vi "Merge Overlay With Image.vi"(6 "Image RGB":T1=refnum, 7 "ROI Cluster":T2={"left annulus"={"Center X"=929, "Center Y"=663, "Inner Radius"=200, "Outer Radius"=405, "Start Angle"=90.0, "End Angle"=180.0}, "right annulus"={"Center X"=929, "Center Y"=663, "Inner Radius"=200, "Outer Radius"=405, "Start Angle"=90.0, "End Angle"=180.0}, "Threshold Range"={"Lower value"=106.82432432432432, "Upper value"=255.0}, "[Avg BG]"=[0, 0, 0, 0, 0, 0, 0, 0, 0, 0, 0, 0, 0, 0, 0, 0, 0, 0, 0, 0, 0, 0, 0, 0, 0, 0, 0, 0, 0, 0, 0, 0], "Number of Sectors"=0, "Left ROI"={"Global Rectangle"=[], "Contours"=[]}, "Right ROI"={"Global Rectangle"=[], "Contours"=[]}, "Left Start Angle Duty Cycle"=0.0, "Left End Angle Duty Cycle"=0.0, "Right End Angle Duty Cycle"=0.0, "Right Start Angle Duty Cycle"=0.0, "[Sector ROIs]"=[], "Consecutive Sector Threshold"=0} {"[Sector ROIs]"."Contours"."Type" items=["No Selection", "Point", "Line", "Rectangle", "Oval", "Polygon", "Freehand Region", "Annulus", "Unused2", "Unused3", "Broken Line", "Freehand Line", "Rotated Rectangle"]; "Right ROI"."Contours"."Type" items=["No Selection", "Point", "Line", "Rectangle", "Oval", "Polygon", "Freehand Region", "Annulus", "Unused2", "Unused3", "Broken Line", "Freehand Line", "Rotated Rectangle"]; "Left ROI"."Contours"."Type" items=["No Selection", "Point", "Line", "Rectangle", "Oval", "Polygon", "Freehand Region", "Annulus", "Unused2", "Unused3", "Broken Line", "Freehand Line", "Rotated Rectangle"]; "Threshold Range"."Upper value" min=0.0 max=255.0 scale=0.0..255.0; "Threshold Range"."Lower value" min=0.0 max=255.0 scale=0.0..255.0; "right annulus"."End Angle" format="%.2f"; "right annulus"."Start Angle" format="%.2f"; "right annulus"."Center X" scale=0.0..1024.0; "left annulus"."End Angle" format="%.2f"; "left annulus"."Start Angle" format="%.2f"; "left annulus"."Center X" scale=0.0..1024.0}, 8 "Error in":errorcluster, 9 "Left Edge":u16, 10 "Right Edge":u16, 11 "Image In":T1=refnum) -> (0 "error out":errorcluster, 3 "Image Out":T1)   [LabVIEW 2013]
uses:
  <vilib>/vision/Image Controls.llb/IMAQ Image.ctl
  Image Processing/Mask ROI Cluster.ctl
  <vilib>/vision/NI_Vision_Development_Module.lvlib
  Common/Timing/Timing Lib.lvlib
panel:
  out "x-y":dbl
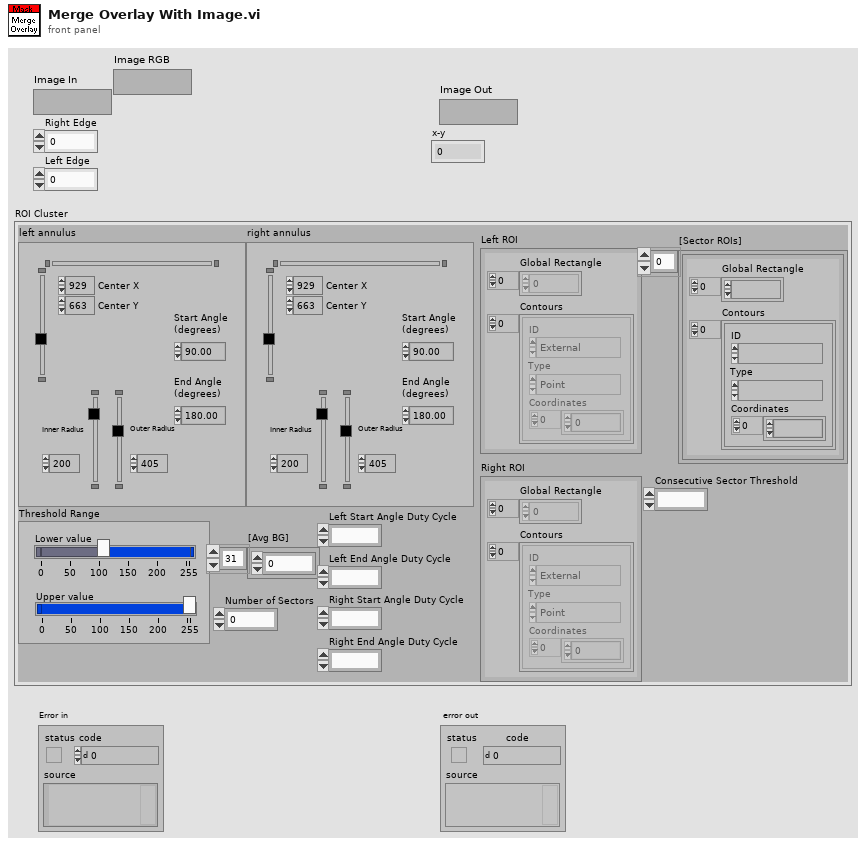
[diagram p1: front panel]
types:
  T1 = typedef "IMAQ Image.ctl" = refnum<image>
  T2 = typedef "Mask ROI Cluster.ctl" = cluster{"left annulus":T3, "right annulus":T3, "Threshold Range":cluster{"Lower value":dbl, "Upper value":dbl}, "[Avg BG]":u8[], "Number of Sectors":u8, "Left ROI":T4, "Right ROI":T4, "Left Start Angle Duty Cycle":fxp<+,8,0>, "Left End Angle Duty Cycle":fxp<+,8,0>, "Right End Angle Duty Cycle":fxp<+,8,0>, "Right Start Angle Duty Cycle":fxp<+,8,0>, "[Sector ROIs]":T4[], "Consecutive Sector Threshold":u8}
  T3 = typedef "IMAQ Circle" = cluster{"Center X":i32, "Center Y":i32, "Inner Radius":i32, "Outer Radius":i32, "Start Angle":dbl, "End Angle":dbl}
  T4 = typedef "ROI Descriptor" = cluster{"Global Rectangle":i32[], "Contours":cluster{"ID":enum32{"External", "Internal"}, "Type":u32, "Coordinates":i32[]}[]}
  T5 = typedef "Image Type" = u32
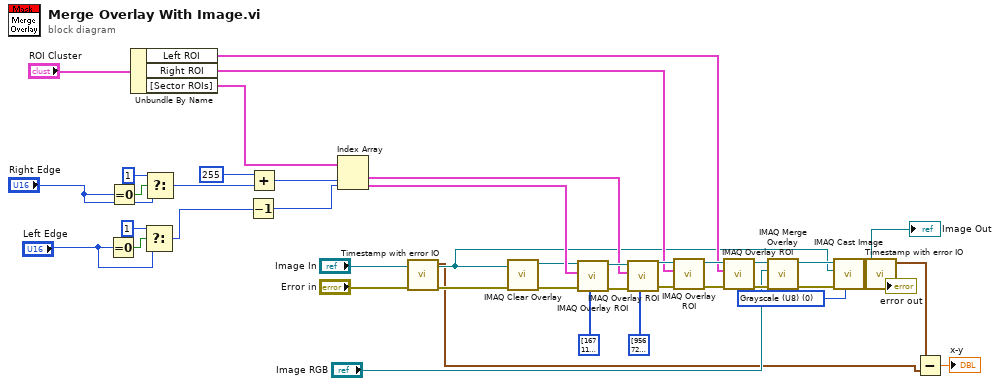
[diagram p0: block diagram]
diagram:
  w10 = T5 0 items=["Grayscale (U8)", "Grayscale (I16)", "Grayscale (SGL)", "Complex (CSG)", "RGB (U32)", "HSL (U32)", "RGB (U64)", "Grayscale (U16)"] ("Image Type")
  n1 = Equal To 0?(x="Left Edge") -> (x = 0?=w20:bool)
  n2 = Equal To 0?(x="Right Edge") -> (x = 0?=w22:bool)
  n3 = Unbundle By Name("ROI Cluster") -> ("Left ROI"=w31:T4, "Right ROI"=w30:T4, "[Sector ROIs]"=w29:T4[])
  n4 = Select(t=u16 1, s=w20, f="Left Edge") -> (s? t:f=w18:u16)
  n5 = Select(t=u16 1, s=w22, f="Right Edge") -> (s? t:f=w19:u16)
  n6 = Decrement(x=w18) -> (x-1=w38:u16)
  n7 = Add(x=u16 255, y=w19) -> (x+y=w39:u16)
  n8 = Index Array(array=w29, index #1=w39, index #2=w38) -> (element #1=w32:T4, element #2=w33:T4)
  n9 = call "Timestamp with error IO.vi"("error in (no error)"="Error in") -> ("error out"=w5:errorcluster, "current time"=w2:timestamp)  [unwired: 9 in]
  n10 = call "IMAQ Clear Overlay"("error in (no error)"=w5, "Image"="Image In") -> ("error out"=w26:errorcluster, "Image Out"=w27:T1)  [unwired: 8 in]
  n11 = call "IMAQ Overlay ROI"("Colors (Green)"=u32[] [16711935], "error in (no error)"=w26, "ROI Descriptor"=w33, "Image"=w27) -> ("error out"=w42:errorcluster, "Image Out"=w41:T1)  [unwired: 6 in]
  n12 = call "IMAQ Overlay ROI"("Colors (Green)"=u32[] [9567230], "error in (no error)"=w42, "ROI Descriptor"=w32, "Image"=w41) -> ("error out"=w34:errorcluster, "Image Out"=w36:T1)  [unwired: 6 in]
  n13 = call "IMAQ Overlay ROI"("error in (no error)"=w34, "ROI Descriptor"=w30, "Image"=w36) -> ("error out"=w37:errorcluster, "Image Out"=w35:T1)  [unwired: 7 in]
  n14 = call "IMAQ Overlay ROI"("error in (no error)"=w37, "ROI Descriptor"=w31, "Image"=w35) -> ("error out"=w14:errorcluster, "Image Out"=w13:T1)  [unwired: 7 in]
  n15 = call "IMAQ Merge Overlay"("error in (no error)"=w14, "Image Dst"="Image RGB", "Image Src"=w13) -> ("error out"=w6:errorcluster, "Image Dst Out"=w9:T1)  [unwired: 7 in]
  n16 = call "IMAQ Cast Image"("Image Type"=w10, "error in (no error)"=w6, "Image Dst"="Image In", "Image Src"=w9) -> ("error out"=w11:errorcluster, "Image Dst Out"=→"Image Out":T1)  [unwired: 6 in]
  n17 = call "Timestamp with error IO.vi"("error in (no error)"=w11) -> ("error out"=→"error out":errorcluster, "current time"=w3:timestamp)  [unwired: 9 in]
  n18 = Subtract(x=w3, y=w2) -> (x-y=→"x-y":dbl)
